vi "Server Close.vi"(8 "error in (no error)":errorcluster, 11 "VisionServerRef in":T1) -> (0 "error out":errorcluster, 3 "VisionServerRef out":T1)   [LabVIEW 2016, in "Vision Server.lvclass"]
uses:
  Vision Server.lvclass
  typedef/Vision Server Ref.ctl
  Vision Server.lvclass/Vision Server.ctl
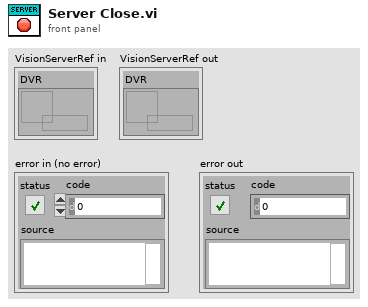
[diagram p1: front panel]
types:
  T1 = typedef "Vision Server.lvclass/Vision Server Ref.ctl" = cluster{"DVR":refnum<data-value>}
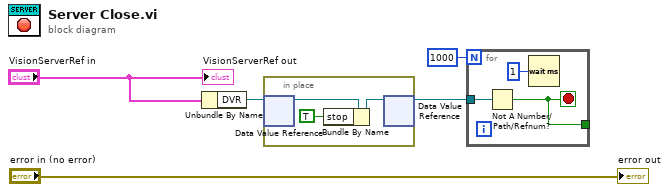
[diagram p0: block diagram]
diagram:
  n1 = Unbundle By Name("VisionServerRef in") -> ("DVR"=w3:refnum<data-value>)
  n2 = in-place {
    n3 = in-place-dvr #1(w3) -> (w8:refnum<class "Vision Server.lvclass">)  [unwired: 1 out]
    n4 = Bundle By Name(cluster=w8, "stop"=TRUE) -> (w7:refnum<class "Vision Server.lvclass">)
    n5 = in-place-dvr #1(w7) -> (w2:refnum<data-value>)  [unwired: 1 out]
  }
  n6 = for {
    N: 1000 -> [_]
    tunnel: w2 -> [w11]
    tunnel: [w9] -> _
    stop <- w9 stop-if-true
    n7 = Not A Number/Path/Refnum?(number/path/refnum=w11) -> (NaN/Path/Refnum?=w9:bool)
    n8 = Wait (ms)(milliseconds to wait=u32 1) -> ()  [unwired: 1 out]
  }
  "error out" <- "error in (no error)"
  "VisionServerRef out" <- "VisionServerRef in"
